vi "Timestamp_equal_to_current_time.vi"(7 "time format string (%c)":string="%c", 8 "error in (no error)":errorcluster, 10 "time stamp":timestamp) -> (0 "error out":errorcluster, 2 "Boolean":bool)   [LabVIEW 2020]
doc: "This VI takes input <b> timestamp </b> and checks if it's equal to current date.<b> Time format string (%c) </b> specifies the format of the comparison (e.g. time format string = %H:%M program compares only hours and minutes). If <b> timestamp </b> is equal to current date the program returns boolean TRUE."
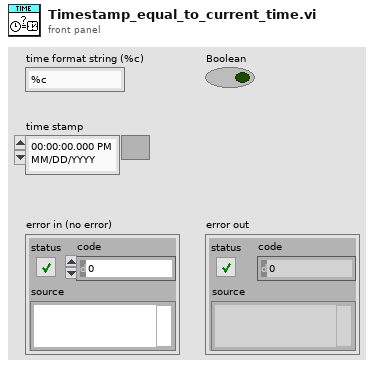
[diagram p1: front panel]
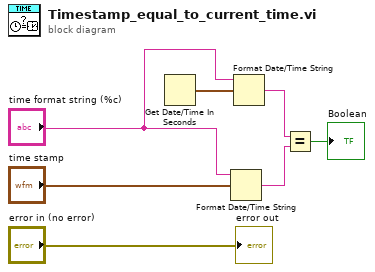
[diagram p0: block diagram]
diagram:
  n1 = Get Date/Time In Seconds() -> (seconds since 1Jan1904=w2:timestamp)
  n2 = Format Date/Time String(time format string (%c)="time format string (%c)", seconds (now)="time stamp") -> (date/time string=w4:string)  [unwired: 1 in]
  n3 = Format Date/Time String(time format string (%c)="time format string (%c)", seconds (now)=w2) -> (date/time string=w3:string)  [unwired: 1 in]
  n4 = Equal?(x=w3, y=w4) -> (x = y?=→"Boolean":bool)
  "error out" <- "error in (no error)"
